vi "Shooter Math.vi"(2 "Time":dbl, 4 "Distance":dbl) -> (0 "Potent":dbl, 1 "Speed":dbl)   [LabVIEW 2012]
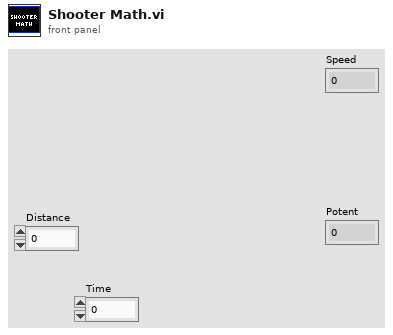
[diagram p1: front panel]
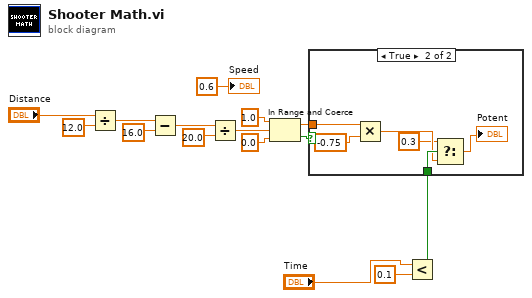
[diagram p0: block diagram]
diagram:
  n1 = Divide(x="Distance", y=12.0) -> (x/y=w13:dbl)
  n2 = Subtract(x=w13, y=16.0) -> (x-y=w11:dbl)
  n3 = Divide(x=w11, y=20.0) -> (x/y=w9:dbl)
  n4 = In Range and Coerce(upper limit=1.0, x=w9, lower limit=0.0) -> (coerced(x)=w5:dbl, In Range?=w6:bool)
  n5 = Less?(x="Time", y=0.1) -> (x < y?=w2:bool)
  n6 = case shown="True" w6 {
    tunnel: w5 -> [_ w21]
    tunnel: w2 -> [_ w19]
    frame False {
    }
    frame True {
      n7 = Multiply(x=w21, y=-0.75) -> (x*y=w18:dbl)
      n8 = Select(t=0.3, s=w19, f=w18) -> (s? t:f=→"Potent":dbl)
    }
  }
  "Speed" <- 0.6 ("y")
